vi "Behaviors and stuff in progress.vi"() -> ()   [LabVIEW 2016]
uses:
  <vilib>/addons/control/pid/NI_PID_pid.lvlib
  <vilib>/addons/control/pid/pid.llb/PID (DBL).vi
  <vilib>/Rock Robotics/WPI/Solenoid/Deprecated/WPI_SolenoidSetBool.vi
  <vilib>/Rock Robotics/WPI/Solenoid/Deprecated/WPI_SolenoidGetBool.vi
  <vilib>/platform/TimedLoop/XDataNode/XDataNode.xnode
  <vilib>/Platform/TimedLoop/XDataNode/nitl_modes.ctl
  <vilib>/Platform/TimedLoop/XDataNode/XDNodeRunTimeDep.lvlib
  <vilib>/Platform/TimedLoop/XDataNode/wakeup.ctl
  <vilib>/Platform/TimedLoop/XDataNode/timing_clust.ctl
  Intake Commands.ctl
  <vilib>/Rock Robotics/SystemInterfaces/DIO/FPGA_DIOPWMChannel.ctl
  <vilib>/Rock Robotics/WPI/PWM/WPI_PWMDeadband.ctl
  <vilib>/Rock Robotics/WPI/MotorControl/WPI_MotorControlType.ctl
  <vilib>/Rock Robotics/WPI/MotorControl/WPI_MotorControlDeviceRef.ctl
panel:
  in  "PID gains 2":T1={"proportional gain (Kc)"=1.0, "integral time (Ti, min)"=0.01, "derivative time (Td, min)"=0.0} {"derivative time (Td, min)" format="%.3f"; "integral time (Ti, min)" format="%.3f"; "proportional gain (Kc)" format="%.3f"}
  in  "Offset":dbl
  in  "Max Throttle":dbl
  in  "Negate":bool
  in  "MotorControlDevRef":T2={"DeviceStatus"={"status"=FALSE, "code"=0, "source"=""}, "Type"=enum."PWM", "PWM"={"PWM Channel"=enum."Invalid", "DeadBand"={"Name"="", "maxPositivePwm"=0, "minPositivePwm"=0, "centerPwm"=0, "maxNegativePwm"=0, "minNegativePwm"=0, "angularRange"=0}}, "CAN"={"Device Number"=0, "SetOutput VI Ref"=variant(enum8{"Percent VBus", "Current", "Speed", "Position", "Voltage"} enum."Percent VBus"), "GetOutput VI Ref"=variant(refnum<k1> refnum), "Enable VI Ref"=variant(dbl 12.0), "Disable VI Ref"=variant(enum8{"Percent VBus", "Speed", "Position", "Slave", "Unchanged / Invalid"} enum."Percent VBus"), "Data"=variant}, "Invert"=FALSE}
  in  "?":T6
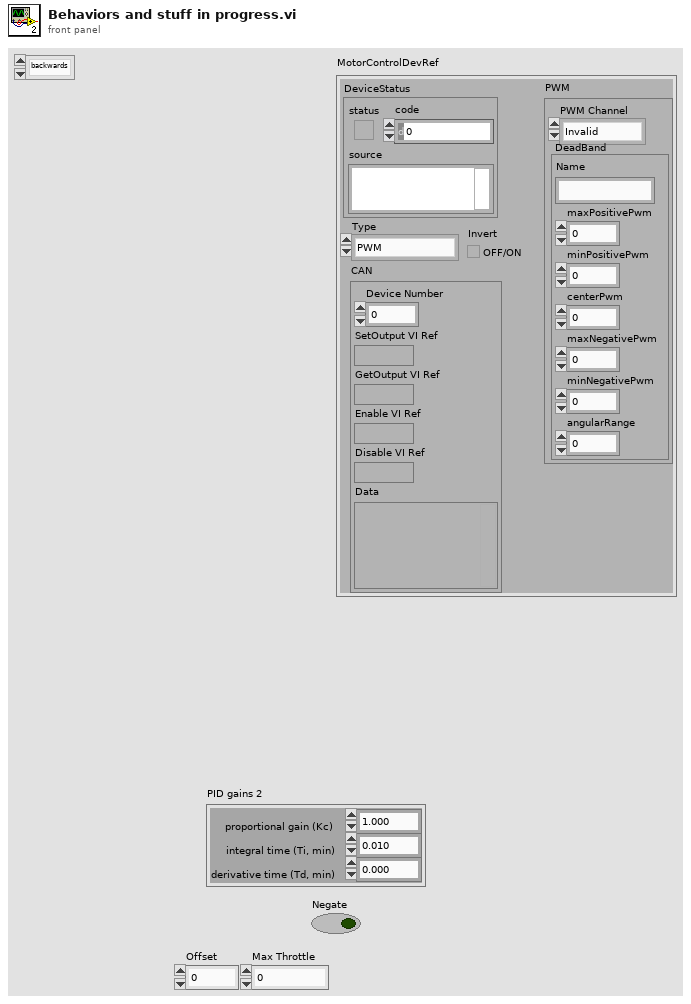
[diagram p1: front panel]
types:
  T1 = cluster{"proportional gain (Kc)":dbl, "integral time (Ti, min)":dbl, "derivative time (Td, min)":dbl}
  T2 = typedef "WPI_MotorControlDeviceRef.ctl" = cluster{"DeviceStatus":errorcluster, "Type":T3, "PWM":cluster{"PWM Channel":T4, "DeadBand":T5}, "CAN":cluster{"Device Number":u8, "SetOutput VI Ref":variant, "GetOutput VI Ref":variant, "Enable VI Ref":variant, "Disable VI Ref":variant, "Data":variant}, "Invert":bool}
  T3 = typedef "WPI_MotorControlType.ctl" = enum16{"PWM", "CAN"}
  T4 = typedef "FPGA_DIOPWMChannel.ctl" = enum8{"PWM 0", "PWM 1", "PWM 2", "PWM 3", "PWM 4", "PWM 5", "PWM 6", "PWM 7", "PWM 8", "PWM 9", "PWM MXP 0", "PWM MXP 1", "PWM MXP 2", "PWM MXP 3", "PWM MXP 4", "PWM MXP 5", "PWM MXP 6", "PWM MXP 7", "PWM MXP 8", "PWM MXP 9", "Invalid"}
  T5 = typedef "WPI_PWMDeadband.ctl" = cluster{"Name":string, "maxPositivePwm":i32, "minPositivePwm":i32, "centerPwm":i32, "maxNegativePwm":i32, "minNegativePwm":i32, "angularRange":u16}
  T6 = typedef "Intake Commands.ctl" = enum16{"backwards", "stop", "forward"}
  T7 = typedef "XDNodeRunTimeDep.lvlib/timing_clust.ctl" = cluster{"Expected End [f-1]":u64, "Actual End [f-1]":u64, "Finished Late? [f-1]":bool, "Expected End [i-1]":u64, "Actual End [i-1]":u64, "Finished Late? [i-1]":bool, "Expected Start [i]":u64, "Actual Start [i]":u64, "Expected Start [f]":u64, "Actual Start [f]":u64, "Source Name":string, "Structure Name":string, "Period":i64, "Deadline":i64, "Offset":i64, "Start":i64, "Priority":i32, "Timeout":i32, "Mode":T8, "Wakeup Reason":T9, "Error":errorcluster, "Source Type":string, "Secondary Source Type":string, "Global End Time":u64, "Global Start Time":u64, "Frame Duration":u64, "Iteration Duration":u64, "Assigned CPU":i32, "I/O Scan Engine Mode":u32}
  T8 = typedef "XDNodeRunTimeDep.lvlib/nitl_modes.ctl" = enum32{"No Change", "Process missed periods, maintain original phase", "Discard missed periods, maintain original phase", "Process missed periods, ignore original phase", "Discard missed periods, ignore original phase"}
  T9 = typedef "XDNodeRunTimeDep.lvlib/wakeup.ctl" = enum32{"Normal", "Aborted", "Asynchronous wakeup", "Timing source error", "Timed loop error", "Timeout"}
  T10 = typedef "WPI_SolenoidDevRef.ctl" = cluster{"DevStatus":errorcluster, "Pneumatics Control Module":u8, "Forward Solenoid Channel":T11, "Reverse Solenoid Channel":T11}
  T11 = typedef "WPI_SolenoidChannel.ctl" = enum8{"Solenoid 0", "Solenoid 1", "Solenoid 2", "Solenoid 3", "Solenoid 4", "Solenoid 5", "Solenoid 6", "Solenoid 7", "Invalid"}
  T12 = typedef "Drive_Code_Bundle.ctl" = cluster{"Sensor Data":T13, "Drive Command rt fifo":refnum<k33>, "Logging Data":refnum<k33>, "PID Update":refnum<notifier>}
  T13 = typedef "Sensor_Cluster.ctl" = cluster{"Gyro Data":cluster{"Gyro RT FIFO":refnum<k33>, "Gyro Current":dbl, "Gyro Hold":dbl}, "Encoder Data":cluster{"Encoder RT FIFO":refnum<k33>, "Encoder Current":dbl, "Encoder Hold":dbl}, "Camera Data":cluster{"Camera RT FIFO":refnum<k33>, "Camera Current":T14}}
  T14 = typedef "Camera_Cluster.ctl" = cluster{" Angle":dbl, "Valid":bool}
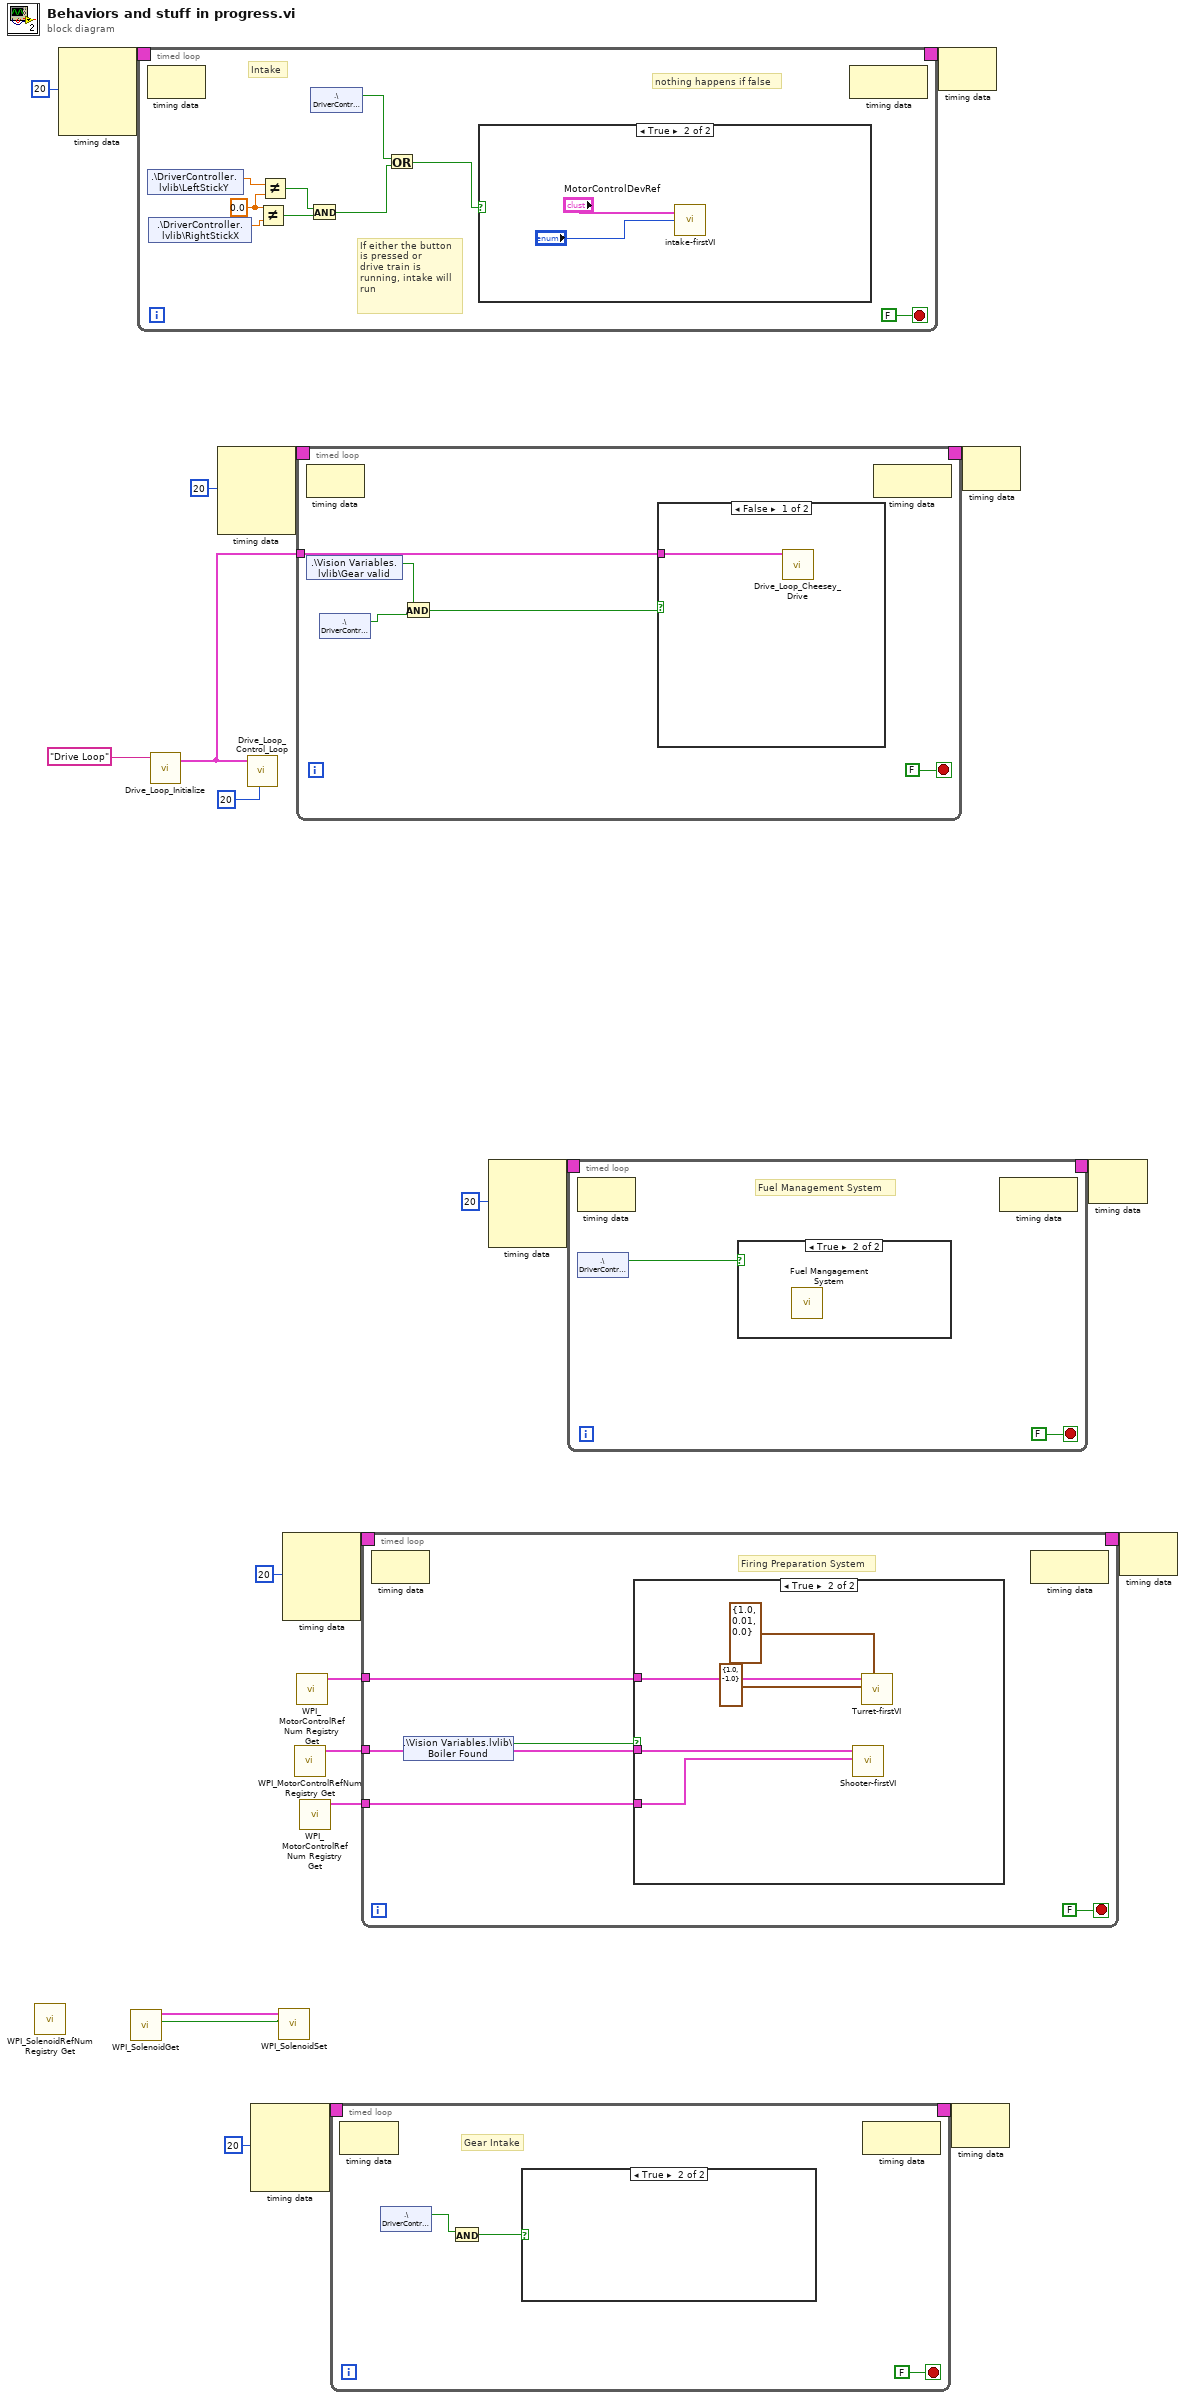
[diagram p0: block diagram]
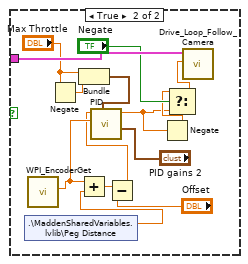
[diagram p3: hidden frame]
diagram:
  n1 = call <vilib>:"WPI_SolenoidRefNum Registry Get.vi"() -> ()  [unwired: 10 in, 2 out]
  n2 = node-c288(i64 20 ("Period")) -> (w7:T7)  [unwired: 3 in]
  n3 = call-poly <vilib>:"WPI_SolenoidGet.vi"() -> ("Value"=w16:bool, "SolenoidDevRef"=w17:T10)  [unwired: 9 in, 1 out]
  n4 = timed-loop {
    timing: w7 -> [_]
    timing-out: [_] -> w6
    stop <- FALSE stop-if-true
    w25 = 0.0 ("x")
    # "Intake"
    # "If either the button \nis pressed or \ndrive train is\nrunning, intake will\nrun"
    # "nothing happens if false"
    n5 = node-c288() -> ()  [unwired: 1 in, 1 out]
    n6 = shared-variable ".\\DriverController.lvlib\\LeftStickY"() -> (w27:dbl)  [unwired: 1 in, 1 out]
    n7 = shared-variable ".\\DriverController.lvlib\\RightStickX"() -> (w26:dbl)  [unwired: 1 in, 1 out]
    n8 = Not Equal?(x=w25, y=w26) -> (x != y?=w29:bool)
    n9 = Not Equal?(x=w27, y=w25) -> (x != y?=w28:bool)
    n10 = And(x=w28, y=w29) -> (x .and. y?=w24:bool)
    n11 = shared-variable ".\\DriverController.lvlib\\A"() -> (w30:bool)  [unwired: 1 in, 1 out]
    n12 = Or(x=w30, y=w24) -> (x .or. y?=w32:bool)
    n13 = case shown="True" w32 {
      frame False {
      }
      frame True {
        n14 = call "intake-firstVI.vi"(0:"?", "MotorControlDevRef"="MotorControlDevRef") -> ()
      }
    }
    n15 = node-c288() -> ()  [unwired: 1 in, 1 out]
  }
  n16 = call <userlib>:"Drive_Loop_Initialize.vi"("Name of drive loop (give it a name!)"="Drive Loop") -> ("Drive Loop Cluster"=w21:T12)  [unwired: 9 in, 1 out]
  n17 = node-c288(i64 20 ("Period")) -> (w9:T7)  [unwired: 3 in]
  n18 = call <userlib>:"Drive_Loop_Control_Loop.vi"("Period \n- Amount of time between iterations of the timed control loop"=i64 20 ("Period \n- Amount of time between iterations of the timed control loop"), "Control Cluster"=w21) -> ()  [unwired: 10 in]
  n19 = node-c288(i64 20 ("Period")) -> (w15:T7)  [unwired: 3 in]
  n20 = call-poly <vilib>:"WPI_SolenoidSet.vi"("Value"=w16, "SolenoidDevRef"=w17) -> ()  [unwired: 8 in, 2 out]
  n21 = node-c288(i64 20 ("Period")) -> (w13:T7)  [unwired: 3 in]
  n22 = call <vilib>:"WPI_MotorControlRefNum Registry Get.vi"() -> ("MotorControlDevRef"=w18:T2)  [unwired: 10 in, 1 out]
  n23 = timed-loop {
    tunnel: w21 -> [w37]
    timing: w9 -> [_]
    timing-out: [_] -> w8
    stop <- FALSE stop-if-true
    n24 = node-c288() -> ()  [unwired: 1 in, 1 out]
    n25 = shared-variable ".\\Vision Variables.lvlib\\Gear valid"() -> (w40:bool)  [unwired: 1 in, 1 out]
    n26 = shared-variable ".\\DriverController.lvlib\\X"() -> (w39:bool)  [unwired: 1 in, 1 out]
    n27 = And(x=w40, y=w39) -> (x .and. y?=w38:bool)
    n28 = case shown="False" w38 {
      tunnel: w37 -> [w44 w58]
      frame False {
        n29 = call <userlib>:"Drive_Loop_Cheesey_Drive.vi"("Drive Loop Cluster"=w44) -> ()  [unwired: 11 in]
      }
      frame True {
        n30 = shared-variable ".\\MaddenSharedVariables.lvlib\\Peg Distance"() -> (w52:dbl)  [unwired: 1 in, 1 out]
        n31 = call <vilib>:"WPI_EncoderGet.vi"() -> ("Distance"=w56:dbl)  [unwired: 6 in, 5 out]
        n32 = Negate(x="Max Throttle") -> (-x=w50:dbl)
        n33 = Bundle("Max Throttle"="Max Throttle", w50) -> (w49:cluster{"Max Throttle":dbl, dbl})  [unwired: 1 in]
        n34 = Add(x=w56, y=w52) -> (x+y=w55:dbl)
        n35 = Subtract(x=w55, y="Offset") -> (x-y=w53:dbl)
        n36 = call-poly <vilib>:"PID.vi"("output range"=w49, "PID gains"="PID gains 2", "process variable"=w56, "setpoint"=w53) -> ("output"=w46:dbl)  [unwired: 6 in, 1 out]
        n37 = Negate(x=w46) -> (-x=w47:dbl)
        n38 = Select(t=w47, s="Negate", f=w46) -> (s? t:f=w45:dbl)
        n39 = call <userlib>:"Drive_Loop_Follow_Camera.vi"("Power Level #6"=w45, "Drive Loop Cluster"=w58) -> ()  [unwired: 10 in]
      }
    }
    n40 = node-c288() -> ()  [unwired: 1 in, 1 out]
  }
  n41 = call <vilib>:"WPI_MotorControlRefNum Registry Get.vi"() -> ("MotorControlDevRef"=w20:T2)  [unwired: 10 in, 1 out]
  n42 = call <vilib>:"WPI_MotorControlRefNum Registry Get.vi"() -> ("MotorControlDevRef"=w19:T2)  [unwired: 10 in, 1 out]
  n43 = timed-loop {
    timing: w15 -> [_]
    timing-out: [_] -> w14
    stop <- FALSE stop-if-true
    # "Gear Intake"
    n44 = node-c288() -> ()  [unwired: 1 in, 1 out]
    n45 = shared-variable ".\\DriverController.lvlib\\X"() -> (w59:bool)  [unwired: 1 in, 1 out]
    n46 = And(x=w59) -> (x .and. y?=w60:bool)  [unwired: 1 in]
    n47 = case shown="True" w60 {
      frame False {
      }
      frame True {
      }
    }
    n48 = node-c288() -> ()  [unwired: 1 in, 1 out]
  }
  n49 = timed-loop {
    tunnel: w20 -> [w66]
    tunnel: w19 -> [w65]
    tunnel: w18 -> [w64]
    timing: w13 -> [_]
    timing-out: [_] -> w12
    stop <- FALSE stop-if-true
    # "Firing Preparation System"
    n50 = node-c288() -> ()  [unwired: 1 in, 1 out]
    n51 = shared-variable ".\\Vision Variables.lvlib\\Boiler Found"() -> (w68:bool)  [unwired: 1 in, 1 out]
    n52 = case shown="True" w68 {
      tunnel: w66 -> [_ w75]
      tunnel: w65 -> [_ w74]
      tunnel: w64 -> [_ w73]
      frame False {
      }
      frame True {
        n53 = call "Shooter-firstVI.vi"("topWheelMotor"=w74, "bottomWheelMotor"=w73) -> ()  [unwired: 9 in, 1 out]
        n54 = call "Turret-firstVI.vi"("PID gains"=T1 {"proportional gain (Kc)"=1.0, "integral time (Ti, min)"=0.01, "derivative time (Td, min)"=0.0}, "output range"=cluster{"output high":dbl, "output low":dbl} {"output high"=1.0, "output low"=-1.0}, "MotorControlDevRef"=w75) -> ()  [unwired: 8 in, 1 out]
      }
    }
    n55 = node-c288() -> ()  [unwired: 1 in, 1 out]
  }
  n56 = node-c288(i64 20 ("Period")) -> (w11:T7)  [unwired: 3 in]
  n57 = timed-loop {
    timing: w11 -> [_]
    timing-out: [_] -> w10
    stop <- FALSE stop-if-true
    # "Fuel Management System"
    n58 = node-c288() -> ()  [unwired: 1 in, 1 out]
    n59 = shared-variable ".\\DriverController.lvlib\\Y"() -> (w76:bool)  [unwired: 1 in, 1 out]
    n60 = case shown="True" w76 {
      frame False {
      }
      frame True {
        n61 = call "Fuel Mangagement System.vi"() -> ()  [unwired: 12 in]
      }
    }
    n62 = node-c288() -> ()  [unwired: 1 in, 1 out]
  }
  n63 = node-c288(w6) -> ()  [unwired: 1 out]
  n64 = node-c288(w14) -> ()  [unwired: 1 out]
  n65 = node-c288(w8) -> ()  [unwired: 1 out]
  n66 = node-c288(w10) -> ()  [unwired: 1 out]
  n67 = node-c288(w12) -> ()  [unwired: 1 out]
